vi "FGV Pre Test Zustandsautomat.vi"(7 "abgebrochen":bool, 10 "Aktion":T1) -> (0 "Tabelle Wertänderung":bool, 1 "Fertig":bool, 2 "Aktion":T1, 3 "Status":string)   [LabVIEW 2020, in "EPA 1065.lvlib" / "Pre-test verification 1065-520.lvlib"]
uses:
  Pre-test verification 1065-520.lvlib
  Aktion FGV Pre Test Zustandsautomat.ctl
  Sprachverwaltung/FGV Aktion Tabelle zerlegen.ctl
  Seiten/CalGas Aufschaltung/FGV CalGas Aktionen.ctl
  Aktion FGV Pre Test Daten.ctl
  Allgemeine VIs/Aktion Test Status.ctl
  Funktionstasten/Zustaende.ctl
  Funktionstasten/Funktionstasten-Aktion.ctl
  PNS/Aktionen FGV Grenzwerte.ctl
  Seiten/CalGas Aufschaltung/Auswahl Aufschaltpunkt.ctl
  Funktionstasten/Funktionstasten.lvlib
  Seiten/FT-IR/FT-IR.lvlib
  Sprachverwaltung/Sprachverwaltung.lvlib
  Seiten/CalGas Aufschaltung/CalGas Aufschaltung.lvlib
  PNS/PNS.lvlib
  EPA 1065.lvlib
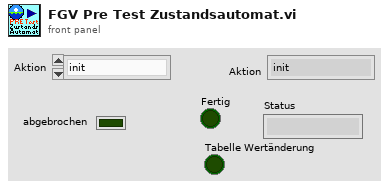
[diagram p1: front panel]
types:
  T1 = typedef "EPA 1065.lvlib/Pre-test verification 1065-520.lvlib/Aktion FGV Pre Test Zustandsautomat.ctl" = enum16{"init", "lesen", "leerlauf", "0-Gas aufschalten", "0-Gas abwarten", "aufzeichnen", "fertig", "abbrechen"}
  T2 = typedef "EPA 1065.lvlib/Aktion Test Status.ctl" = enum16{"init", "lesen", "prüfen", "Interference 366", "Interference 375", "Chiller läuft", "Drift läuft", "Pre Test läuft", "FID Optimization läuft", "FID Interference läuft"}
  T3 = typedef "EPA 1065.lvlib/Pre-test verification 1065-520.lvlib/Aktion FGV Pre Test Daten.ctl" = enum16{"lesen", "Konfig Daten", "PDF einstellen", "laden", "speichern", "Werte schreiben", "Auswerten"}
  T4 = typedef "CalGas Aufschaltung.lvlib/FGV CalGas Aktionen.ctl" = enum16{"lesen", "Analysator Auswahl", "Def.CalGas", "Aufschaltung CalGas", "laden", "speichern", "KAL extrahieren"}
  T5 = typedef "Sprachverwaltung.lvlib/FGV Aktion Tabelle zerlegen.ctl" = enum16{"laden", "vereinzeln", "speichern"}
  T6 = typedef "Funktionstasten.lvlib/Funktionstasten-Aktion.ctl" = enum16{"Initialisieren", "Zustand setzen", "Taste gedrückt", "Fehler speichern", "Lesen", "Manuell", "Remote", "Bitparallel", "Samplepoint", "Zeit Prüfen", "reset Umschalten"}
  T7 = typedef "Funktionstasten.lvlib/Zustaende.ctl" = enum16{"Standby", "Pause", "Eco", "Messen", "Kalibrieren", "Spülen Filter", "Spülen Leitung", "Umgebungsluft", "0-Gas", "Cal-Gas", "CG zu PNS", "-------------", "Init 1", "Init 2", "Init 3", "Init 4", "Messen vorbereiten", "Messen durchführen", "Exit"}
  T8 = typedef "CalGas Aufschaltung.lvlib/Auswahl Aufschaltpunkt.ctl" = enum16{"über Filterblock", "Analysator direkt", "über PNS", "Entnahme", "Gasdivider"}
  T9 = typedef "PNS.lvlib/Aktionen FGV Grenzwerte.ctl" = enum16{"lesen", "Grenzw. schreiben", "Anweisungscode", "IP-Adresse", "laden", "speichern", "Anweisungscode vorgeben"}
  T10 = typedef "EPA 1065.lvlib/Pre-test verification 1065-520.lvlib/Pre Konfig Daten.ctl" = cluster{"Bearbeiter:":string, "Messgerät:":string, "Seriennummer:":string, "Modus":T11, "Pfad:":path, "Textname:":string, "N2 Aufschaltzeit:":dbl, "Flow weighted mean:":dbl}
  T11 = typedef "EPA 1065.lvlib/Pre-test verification 1065-520.lvlib/Modus Pre Test.ctl" = u16
  T12 = typedef "CalGas Aufschaltung.lvlib/Aufschaltung CalGas.ctl" = cluster{"Kalibriergas":T13, "Aufschaltpunkt":T8, "Analysator":T14}
  T13 = typedef "Auswahlfeld.ctl" = u16
  T14 = typedef "CalGas Aufschaltung.lvlib/Auswahl Analysator.ctl" = enum16{"FT-IR", "FID", "PMA", "PMA/FID/FT-IR"}
  T15 = typedef "EPA 1065.lvlib/Pre-test verification 1065-520.lvlib/Pre Werte.ctl" = cluster{"THC Wert":dbl, "Berechnetes Limit":dbl, "Bestanden":bool}
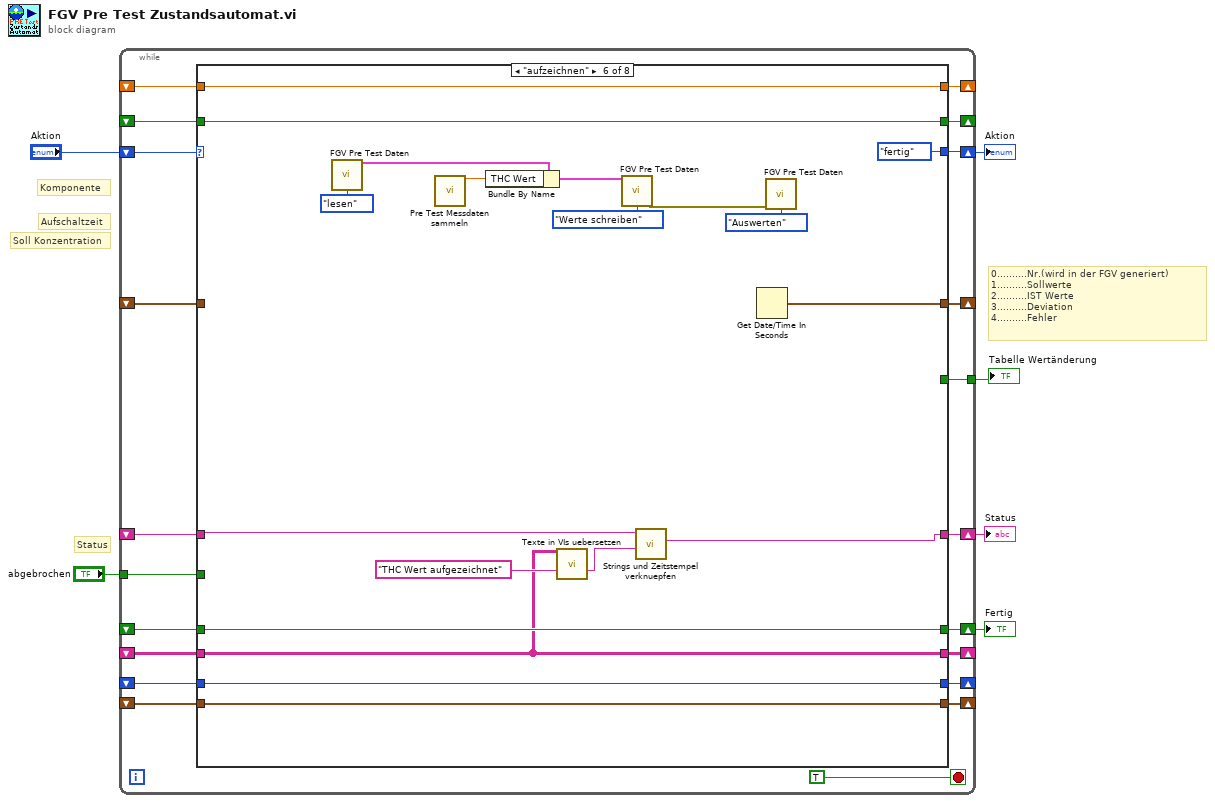
[diagram p0: block diagram]
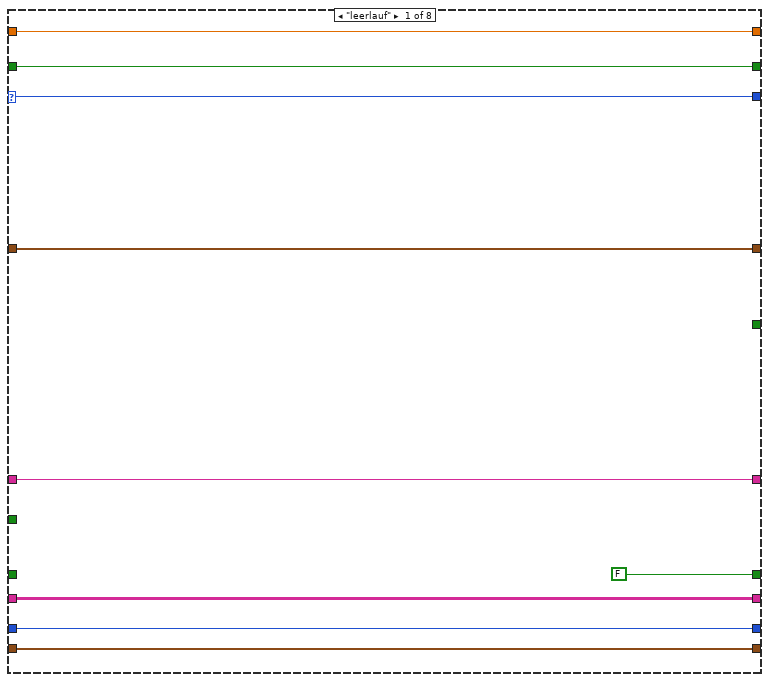
[diagram p2: hidden frame]
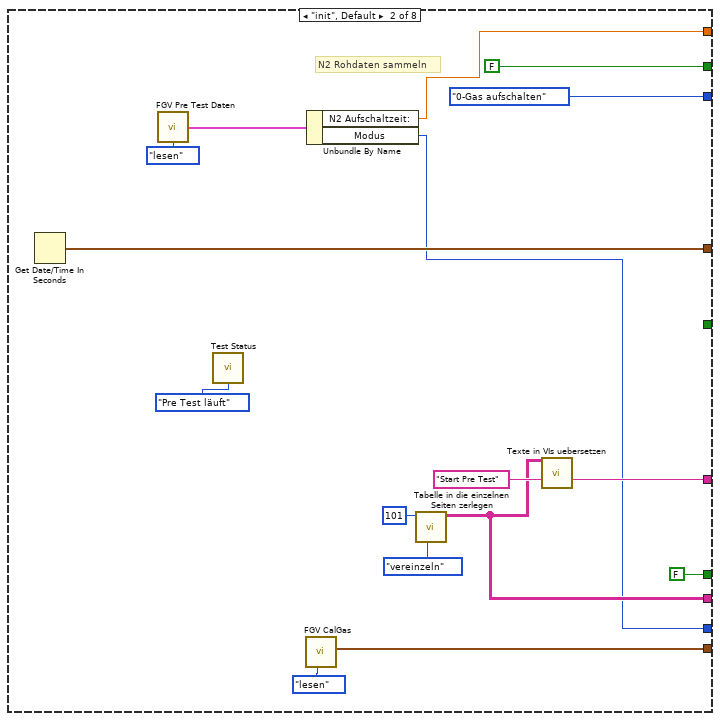
[diagram p3: hidden frame]
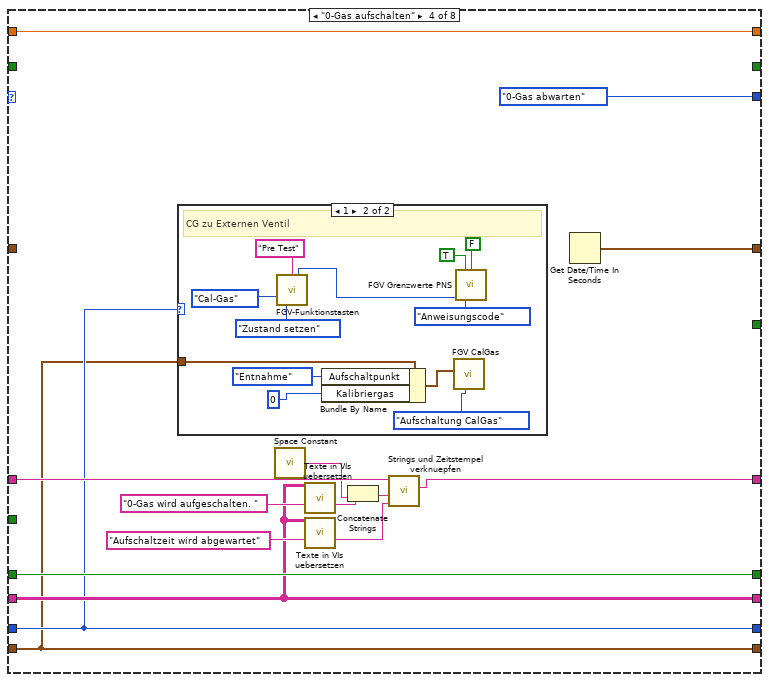
[diagram p5: hidden frame]
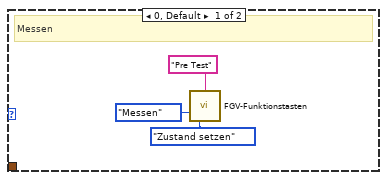
[diagram p6: hidden frame]
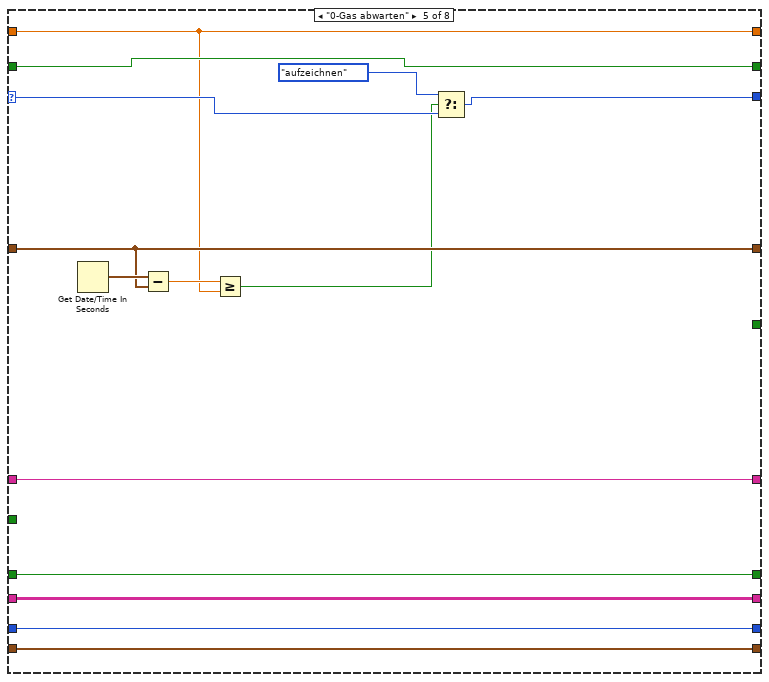
[diagram p7: hidden frame]
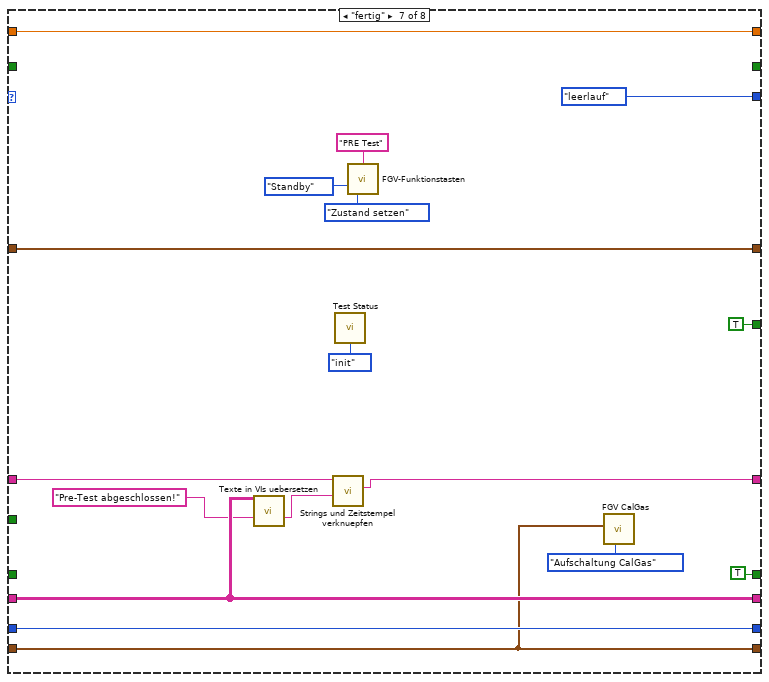
[diagram p8: hidden frame]
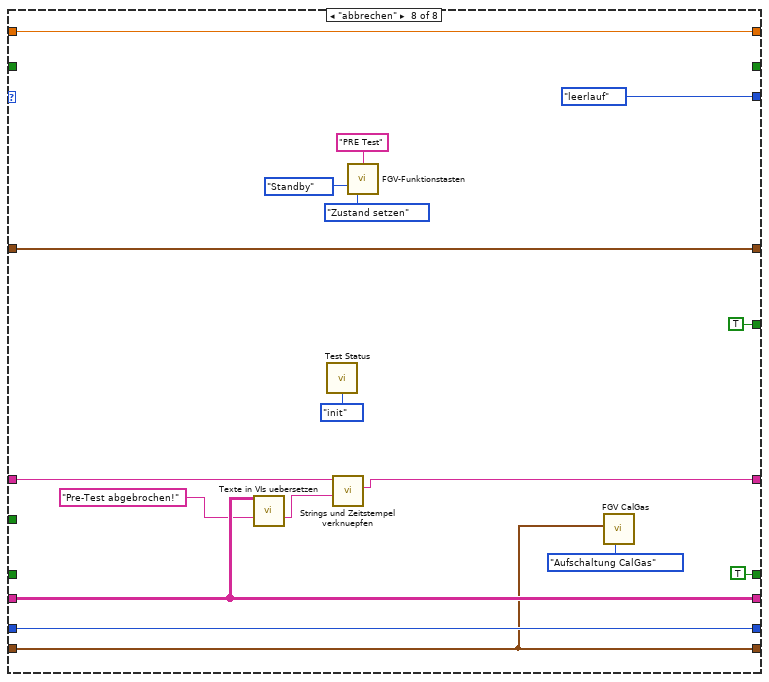
[diagram p9: hidden frame]
diagram:
  # "0..........Nr.(wird in der FGV generiert)\n1..........Sollwerte\n2..........IST Werte\n3..........Deviation\n4..........Fehler"
  # "Status"
  # "Soll Konzentration"
  # "Aufschaltzeit"
  # "Komponente"
  n1 = while {
    shift-right: [w26] -> _
    shift-left: _ -> [w25]
    shift-right: [w24] -> w5
    shift-left: "Aktion" -> [w7]
    shift-right: [w23] -> w4
    shift-left: _ -> [w22]
    tunnel: "abgebrochen" -> [w21]
    shift-right: [w20] -> w2
    shift-left: _ -> [w19]
    shift-right: [w18] -> _
    shift-left: _ -> [w17]
    shift-right: [w16] -> _
    shift-left: _ -> [w15]
    shift-right: [w14] -> _
    shift-left: _ -> [w13]
    shift-right: [w12] -> _
    shift-left: _ -> [w11]
    tunnel: [w10] -> w1
    shift-right: [w9] -> _
    shift-left: _ -> [w8]
    stop <- TRUE stop-if-true
    n2 = case shown="\"aufzeichnen\"" w7 {
      selector: w7 -> [w35 _ w53 _ w102 _ _ _]
      tunnel: [w34 w51 w61 w76 w104 w124 w141 w158] -> w26
      tunnel: w25 -> [w34 _ w61 _ w104 _ w141 w158]
      tunnel: [w35 Aktion_FGV_Pre_Test_Zustandsautomat."0-Gas aufschalten" ("Aktion") w53 Aktion_FGV_Pre_Test_Zustandsautomat."0-Gas abwarten" ("Aktion") w99 Aktion_FGV_Pre_Test_Zustandsautomat."fertig" ("Aktion") Aktion_FGV_Pre_Test_Zustandsautomat."leerlauf" ("Aktion") Aktion_FGV_Pre_Test_Zustandsautomat."leerlauf" ("Aktion")] -> w24
      tunnel: [w33 w47 w60 w73 w98 w106 w139 w156] -> w23
      tunnel: w22 -> [w33 _ w60 w74 w98 w108 w140 w157]
      tunnel: w21 -> [_ _ _ _ _ _ _ _]
      tunnel: [FALSE ("abgebrochen") FALSE ("abgebrochen") w59 w72 w97 w123 TRUE ("abgebrochen") TRUE ("abgebrochen")] -> w20
      tunnel: w19 -> [_ _ w59 w72 w97 w123 _ _]
      tunnel: [w32 w46 w58 w68 w96 w107 w134 w151] -> w18
      tunnel: w17 -> [w32 _ w58 w68 w96 w107 w134 w151]
      tunnel: [w36 FALSE w57 _ w95 w122 _ _] -> w16
      tunnel: w15 -> [w36 _ w57 _ w95 w122 _ _]
      tunnel: [w30 w42 w56 w63 w94 w121 w130 w147] -> w14
      tunnel: w13 -> [w30 _ w56 w63 w94 w121 w130 w147]
      tunnel: [w29 w41 w55 w64 w93 w120 w132 w149] -> w12
      tunnel: w11 -> [w29 _ w55 w64 w93 w120 w132 w149]
      tunnel: [_ _ _ _ _ _ TRUE ("Tabelle Wertänderung") TRUE ("Tabelle Wertänderung")] -> w10
      tunnel: [w28 w40 w54 w62 w92 w119 w128 w145] -> w9
      tunnel: w8 -> [w28 _ w54 w62 w92 w119 w128 w145]
      frame "leerlauf" {
      }
      frame "init", Default {
        # "N2 Rohdaten sammeln"
        n3 = Get Date/Time In Seconds() -> (seconds since 1Jan1904=w51:timestamp)
        n4 = call "FGV Pre Test Daten.vi"("Aktion"=Aktion_FGV_Pre_Test_Daten."lesen") -> ("T90 Konfig Daten 2"=w38:T10)  [unwired: 11 in, 3 out]
        n5 = call "Test Status.vi"("Aktion"=Aktion_Test_Status."Pre Test läuft") -> ()  [unwired: 11 in, 4 out]
        n6 = call "FGV CalGas.vi"("Aktionen"=FGV_CalGas_Aktionen."lesen") -> ("Aufschaltung CalGas"=w42:T12)  [unwired: 6 in, 4 out]
        n7 = Unbundle By Name(w38) -> ("N2 Aufschaltzeit:"=w40:dbl, "Modus"=w41:T11)
        n8 = call "Tabelle in die einzelnen Seiten zerlegen.vi"("Aktion"=FGV_Aktion_Tabelle_zerlegen."vereinzeln", "Index (Seite)"=101) -> ("Sprachliste"=w46:string[][])  [unwired: 7 in, 2 out]
        n9 = call "Texte in VIs uebersetzen.vi"("Sprachliste"=w46, "String zum Übersetzen"="Start Pre Test") -> ("String zum Übersetzen"=w47:string)  [unwired: 9 in, 4 out]
      }
      frame "lesen" {
      }
      frame "0-Gas aufschalten" {
        n10 = case shown="1" w64 {
          tunnel: w63 -> [_ w83]
          frame 0, Default {
            # "Messen"
            n11 = call "FGV-Funktionstasten.vi"("Herkunft"="Pre Test", "Zustand"=Zustaende."Messen", "Aktion"=Funktionstasten-Aktion."Zustand setzen") -> ()  [unwired: 5 in, 8 out]
          }
          frame 1 {
            # "CG zu Externen Ventil"
            n12 = call "FGV-Funktionstasten.vi"("Herkunft"="Pre Test", "Zustand"=Zustaende."Cal-Gas", "Aktion"=Funktionstasten-Aktion."Zustand setzen") -> ("Samplepoint"=w85:u16)  [unwired: 5 in, 7 out]
            n13 = Bundle By Name(cluster=w83, "Aufschaltpunkt"=Auswahl_Aufschaltpunkt."Entnahme", "Kalibriergas"=0) -> (w82:T12)
            n14 = call "FGV CalGas.vi"("Aktionen"=FGV_CalGas_Aktionen."Aufschaltung CalGas", "Aufschaltung CalGas"=w82) -> ()  [unwired: 5 in, 5 out]
            n15 = call "FGV Grenzwerte PNS.vi"("T90"=TRUE ("T90 lüften"), "T90 lüften"=FALSE, "Samplepoint"=w85, "Aktionen FGV Grenzwerte"=Aktionen_FGV_Grenzwerte."Anweisungscode") -> ()  [unwired: 9 in, 3 out]
          }
        }
        n16 = call <vilib>:"Space Constant.vi"() -> ("String"=w66:string)
        n17 = call "Texte in VIs uebersetzen.vi"("Sprachliste"=w68, "String zum Übersetzen"="0-Gas wird aufgeschalten. " ("String 1 hinzufügen")) -> ("String zum Übersetzen"=w67:string)  [unwired: 9 in, 4 out]
        n18 = call "Texte in VIs uebersetzen.vi"("Sprachliste"=w68, "String zum Übersetzen"="Aufschaltzeit wird abgewartet" ("String 2 hinzufügen")) -> ("String zum Übersetzen"=w70:string)  [unwired: 9 in, 4 out]
        n19 = Concatenate Strings(w67, w66) -> (w65:string)
        n20 = call "Strings und Zeitstempel verknuepfen.vi"("String 2 hinzufügen"=w70, "String 1 hinzufügen"=w65, "Eingagns String"=w74) -> ("Verknüpfter String"=w73:string)  [unwired: 8 in]
        n21 = Get Date/Time In Seconds() -> (seconds since 1Jan1904=w76:timestamp)
      }
      frame "0-Gas abwarten" {
        n22 = Get Date/Time In Seconds() -> (seconds since 1Jan1904=w105:timestamp)
        n23 = Subtract(x=w105, y=w104) -> (x-y=w103:dbl)
        n24 = Greater Or Equal?(x=w103, y=w92) -> (x >= y?=w101:bool)
        n25 = Select(t=Aktion_FGV_Pre_Test_Zustandsautomat."aufzeichnen", s=w101, f=w102) -> (s? t:f=w99:T1)
      }
      frame "aufzeichnen" {
        n26 = call "FGV Pre Test Daten.vi"("Aktion"=Aktion_FGV_Pre_Test_Daten."lesen") -> ("Daten/Ergebnisse"=w116:T15)  [unwired: 11 in, 3 out]
        n27 = call "Pre Test Messdaten sammeln.vi"() -> ("Messdaten"=w114:sgl)  [unwired: 14 in, 1 out]
        n28 = Bundle By Name(cluster=w116, "THC Wert"=w114) -> (w115:T15)
        n29 = call "Texte in VIs uebersetzen.vi"("Sprachliste"=w107, "String zum Übersetzen"="THC Wert aufgezeichnet" ("String 1 hinzufügen")) -> ("String zum Übersetzen"=w109:string)  [unwired: 9 in, 4 out]
        n30 = call "FGV Pre Test Daten.vi"("Daten/Ergebnisse"=w115, "Aktion"=Aktion_FGV_Pre_Test_Daten."Werte schreiben") -> ("error out"=w112:errorcluster)  [unwired: 10 in, 3 out]
        n31 = call "Strings und Zeitstempel verknuepfen.vi"("String 1 hinzufügen"=w109, "Eingagns String"=w108) -> ("Verknüpfter String"=w106:string)  [unwired: 9 in]
        n32 = Get Date/Time In Seconds() -> (seconds since 1Jan1904=w124:timestamp)
        n33 = call "FGV Pre Test Daten.vi"("error in (no error)"=w112, "Aktion"=Aktion_FGV_Pre_Test_Daten."Auswerten") -> ()  [unwired: 10 in, 4 out]
      }
      frame "fertig" {
        n34 = call "Texte in VIs uebersetzen.vi"("Sprachliste"=w134, "String zum Übersetzen"="Pre-Test abgeschlossen!" ("String 1 hinzufügen")) -> ("String zum Übersetzen"=w126:string)  [unwired: 9 in, 4 out]
        n35 = call "Strings und Zeitstempel verknuepfen.vi"("String 1 hinzufügen"=w126, "Eingagns String"=w140) -> ("Verknüpfter String"=w139:string)  [unwired: 9 in]
        n36 = call "Test Status.vi"("Aktion"=Aktion_Test_Status."init") -> ()  [unwired: 11 in, 4 out]
        n37 = call "FGV-Funktionstasten.vi"("Herkunft"="PRE Test", "Zustand"=Zustaende."Standby", "Aktion"=Funktionstasten-Aktion."Zustand setzen") -> ()  [unwired: 5 in, 8 out]
        n38 = call "FGV CalGas.vi"("Aktionen"=FGV_CalGas_Aktionen."Aufschaltung CalGas", "Aufschaltung CalGas"=w130) -> ()  [unwired: 5 in, 5 out]
      }
      frame "abbrechen" {
        n39 = call "Texte in VIs uebersetzen.vi"("Sprachliste"=w151, "String zum Übersetzen"="Pre-Test abgebrochen!" ("String 1 hinzufügen")) -> ("String zum Übersetzen"=w143:string)  [unwired: 9 in, 4 out]
        n40 = call "Test Status.vi"("Aktion"=Aktion_Test_Status."init") -> ()  [unwired: 11 in, 4 out]
        n41 = call "Strings und Zeitstempel verknuepfen.vi"("String 1 hinzufügen"=w143, "Eingagns String"=w157) -> ("Verknüpfter String"=w156:string)  [unwired: 9 in]
        n42 = call "FGV-Funktionstasten.vi"("Herkunft"="PRE Test", "Zustand"=Zustaende."Standby", "Aktion"=Funktionstasten-Aktion."Zustand setzen") -> ()  [unwired: 5 in, 8 out]
        n43 = call "FGV CalGas.vi"("Aktionen"=FGV_CalGas_Aktionen."Aufschaltung CalGas", "Aufschaltung CalGas"=w147) -> ()  [unwired: 5 in, 5 out]
      }
    }
  }
  "Aktion" <- w5
  "Status" <- w4
  "Fertig" <- w2
  "Tabelle Wertänderung" <- w1
